vi "setUp.vi"(8 "error in (no error)":errorcluster, 11 "reference in":refnum<class "BM Filters.lvclass">) -> (0 "error out":errorcluster, 3 "reference out":refnum<class "BM Filters.lvclass">)   [LabVIEW 2016, in "BM Filters.lvclass"]
doc: "setUp runs prior to the test method during test execution. Use this method to initialize any object data required by your tests."
uses:
  BM Filters.lvclass
  <vilib>/addons/_JKI Toolkits/VI Tester/TestCase.llb/TestCase.lvclass
  D:/SVN/Products/SLSC/Multichannel 1553 Module/Software/Source Code/Driver (Windows)/Unit Tests/1553 Test/1553 Test.lvclass
  D:/Programs/National Instruments/LabVIEW 2016/vi.lib/addons/_JKI Toolkits/VI Tester/TestCase.llb/TestCase.lvclass
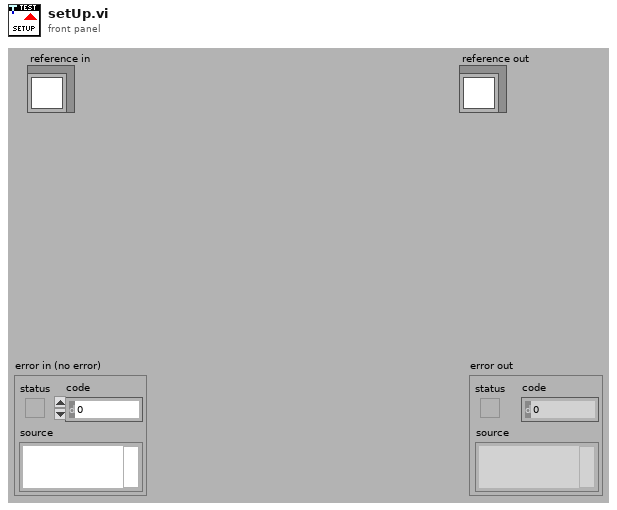
[diagram p1: front panel]
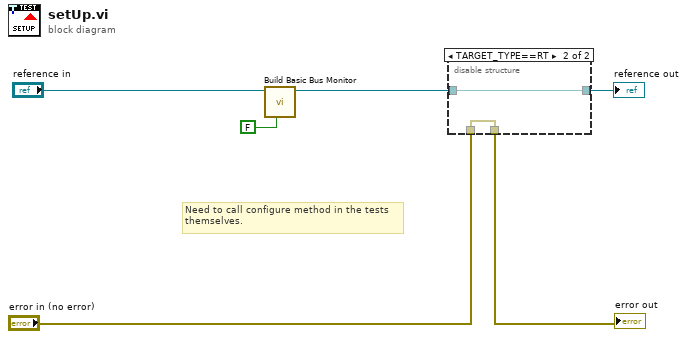
[diagram p0: block diagram]
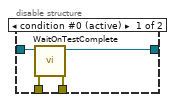
[diagram p2: hidden frame]
diagram:
  # "Need to call configure method in the tests\nthemselves."
  n1 = call-dynamic "Build Basic Bus Monitor.vi"("48-bit Time Tag"=FALSE, "1553 Test in"="reference in") -> ("1553 Test out"=w1:refnum<class "BM Filters.lvclass">)  [unwired: 8 in, 1 out]
  n2 = disable-structure shown="TARGET_TYPE==RT" {
    disable-tunnel: "error in (no error)" -> [w10 w11]
    disable-tunnel: [w9 w11] -> w5
    disable-tunnel: [w8 w12] -> w4
    disable-tunnel: w1 -> [w7 w12]
    frame condition #0 (active) {
      n3 = call <vilib>:"WaitOnTestComplete.vi"("error in (no error)"=w10, "TestCase in"=w7) -> ("error out"=w9:errorcluster, "TestCase out"=w8:refnum<class "BM Filters.lvclass">)  [unwired: 8 in]
    }
    frame condition #1 {
    }
  }
  "error out" <- w5
  "reference out" <- w4
